vi "Sort References By Type.vi"(10 "Controls to Register":refnum<vi>[](array[refnum])) -> (2 "Controls":T1)   [LabVIEW 2019, in "AutoRegistration.lvlib" / "AutoRegistration.lvclass"]
doc: "<License>\nCopyright © 2020 Tymphany, LLC | All rights reserved\nwww.Tymphany.com\nHuijun <Huijun.Guo@Tymphany.com>\n</License>"
uses:
  <vilib>/gpm_packages/@cs/mva-viewable/Source/ActorEvents/AutoRegistration/AutoRegistration.lvclass
  <vilib>/gpm_packages/@cs/mva-viewable/Source/ActorEvents/AutoRegistration/Registration References.ctl
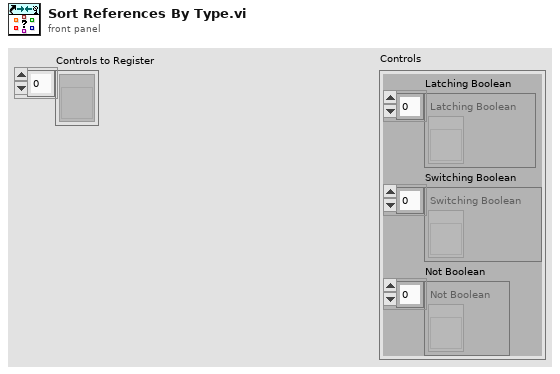
[diagram p1: front panel]
types:
  T1 = typedef "AutoRegistration.lvlib/AutoRegistration.lvclass/Registration References.ctl" = cluster{"Latching Boolean":refnum<vi>[], "Switching Boolean":refnum<vi>[], "Not Boolean":refnum<vi>[]}
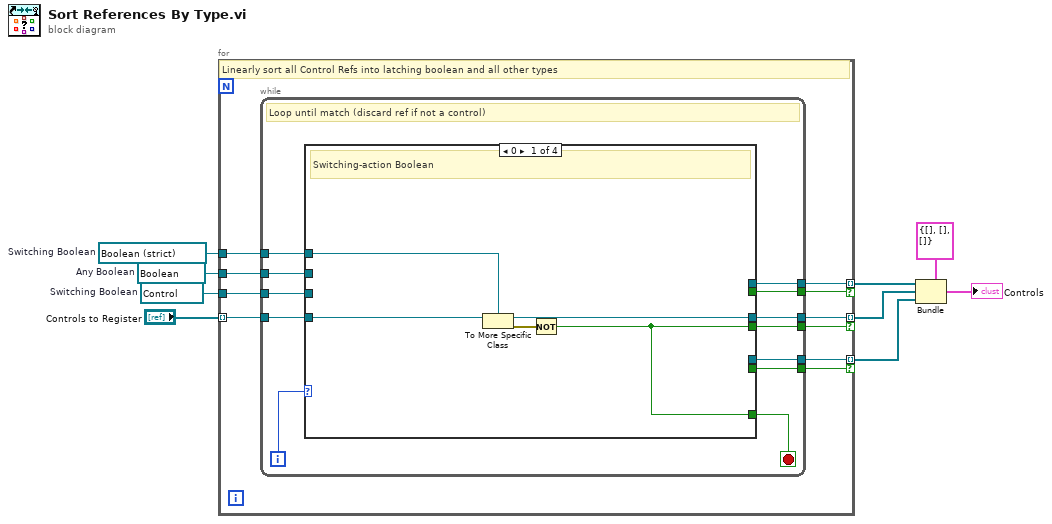
[diagram p0: block diagram]
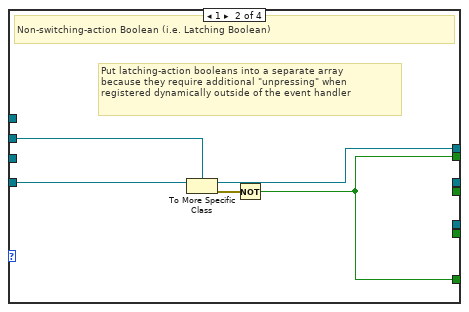
[diagram p2: hidden frame]
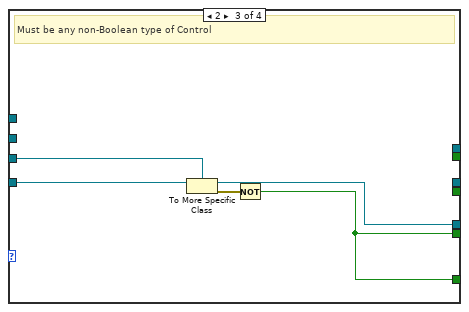
[diagram p3: hidden frame]
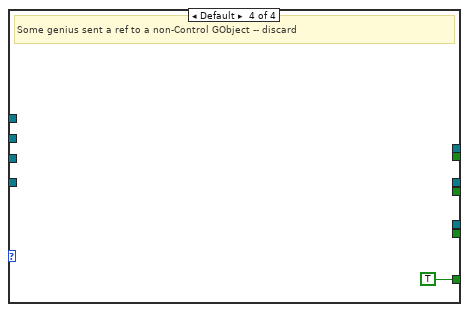
[diagram p4: hidden frame]
diagram:
  w2 = refnum<vi> refnum  # Switching Boolean
  w7 = refnum<vi> refnum  # Switching Boolean
  w8 = refnum<vi> refnum  # Any Boolean
  n1 = for {
    tunnel: "Controls to Register" -> [w13] mode=indexing
    tunnel: w8 -> [w19]
    tunnel: w7 -> [w18]
    tunnel: [w17] -> w6 mode=indexing if=w14
    tunnel: [w16] -> w5 mode=indexing if=w15
    tunnel: w2 -> [w12]
    tunnel: [w11] -> w1 mode=indexing if=w10
    # "Linearly sort all Control Refs into latching boolean and all other types"
    n2 = while {
      tunnel: [w27] -> w15
      tunnel: [w26] -> w14
      tunnel: w13 -> [w25]
      tunnel: w18 -> [w30]
      tunnel: [w29] -> w17
      tunnel: w19 -> [w31]
      tunnel: [w28] -> w16
      tunnel: w12 -> [w22]
      tunnel: [w21] -> w11
      tunnel: [w20] -> w10
      i -> [w23]
      stop <- w24 stop-if-true
      # "Loop until match (discard ref if not a control)"
      n3 = case shown="0" w23 {
        tunnel: w31 -> [_ w41 _ _]
        tunnel: w30 -> [w36 _ _ _]
        tunnel: [_ w38 _ _] -> w29
        tunnel: [w33 _ _ _] -> w28
        tunnel: [w32 _ _ _] -> w27
        tunnel: [_ w37 _ _] -> w26
        tunnel: w25 -> [w34 w39 w45 _]
        tunnel: [w32 w37 w42 TRUE] -> w24
        tunnel: w22 -> [_ _ w44 _]
        tunnel: [_ _ w43 _] -> w21
        tunnel: [_ _ w42 _] -> w20
        frame 0 {
          # "Switching-action Boolean"
          n4 = To More Specific Class(target class=w36, reference=w34) -> (specific class reference=w33:refnum<vi>, error out=w35:errorcluster)  [unwired: 1 in]
          n5 = Not(x=w35) -> (.not. x?=w32:bool)
        }
        frame 1 {
          # "Put latching-action booleans into a separate array\nbecause they require additional \"unpressing\" when\nregistered dynamically outside of the event handler"
          # "Non-switching-action Boolean (i.e. Latching Boolean)"
          n6 = To More Specific Class(target class=w41, reference=w39) -> (specific class reference=w38:refnum<vi>, error out=w40:errorcluster)  [unwired: 1 in]
          n7 = Not(x=w40) -> (.not. x?=w37:bool)
        }
        frame 2 {
          # "Must be any non-Boolean type of Control"
          n8 = To More Specific Class(target class=w44, reference=w45) -> (specific class reference=w43:refnum<vi>, error out=w46:errorcluster)  [unwired: 1 in]
          n9 = Not(x=w46) -> (.not. x?=w42:bool)
        }
        frame Default {
          # "Some genius sent a ref to a non-Control GObject -- discard"
        }
      }
    }
  }
  n10 = Bundle(cluster=T1 {"Latching Boolean"=[], "Switching Boolean"=[], "Not Boolean"=[]} ("Controls"), "Latching Boolean"=w6, "Switching Boolean"=w5, "Not Boolean"=w1) -> (→"Controls":T1)
